vi "ep_Add Parameters of 1st Harmonic.vi"(8 "phase delays in [deg]":dbl[][][](array[numeric]), 9 "gains in":dbl[][][](array[numeric]), 10 "frequencies to calibrate in [Hz]":dbl[](array[numeric]), 11 "norminal frequency [Hz]":dbl) -> (0 "phase delays out [deg]":dbl[][][](array[numeric]), 1 "gains out":dbl[][][](array[numeric]), 2 "frequencies to calibrate out [Hz]":dbl[](array[numeric]))   [LabVIEW 2012]
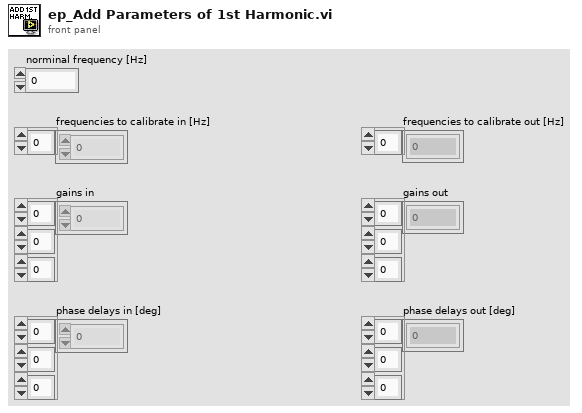
[diagram p1: front panel]
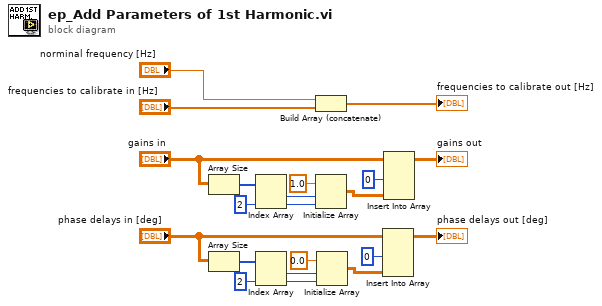
[diagram p0: block diagram]
diagram:
  n1 = Array Size(array="gains in") -> (size(s)=w14:i32[])
  n2 = Array Size(array="phase delays in [deg]") -> (size(s)=w13:i32[])
  n3 = Index Array(array=w14, index #2=2 ("index")) -> (element #1=w12:i32, element #2=w11:i32)  [unwired: 1 in]
  n4 = Index Array(array=w13, index #2=2 ("index")) -> (element #1=w7:i32, element #2=w8:i32)  [unwired: 1 in]
  n5 = Build Array (concatenate)("norminal frequency [Hz]", "frequencies to calibrate in [Hz]") -> (→"frequencies to calibrate out [Hz]":dbl[])
  n6 = Initialize Array(1.0 ("element"), w12, w11) -> (w4:dbl[][])
  n7 = Initialize Array(0.0 ("element"), w7, w8) -> (w3:dbl[][])
  n8 = Insert Into Array(array="phase delays in [deg]", index (dim 1)=0 ("disabled index (row)"), new element=w3) -> (→"phase delays out [deg]":dbl[][][])  [unwired: 2 in]
  n9 = Insert Into Array(array="gains in", index (dim 1)=0 ("disabled index (row)"), new element=w4) -> (→"gains out":dbl[][][])  [unwired: 2 in]
